vi "Write Scale.vi"(8 "error in (no error)":errorcluster, 10 "Scale":dbl, 11 "Multiplexer configuration in":refnum<class "Multiplexer configuration.lvclass">) -> (0 "error out":errorcluster, 3 "Multiplexer configuration out":refnum<class "Multiplexer configuration.lvclass">)   [LabVIEW 2021, in "Multiplexer configuration.lvclass"]
uses:
  Multiplexer configuration.lvclass
  Multiplexer configuration.lvclass/Multiplexer configuration.ctl
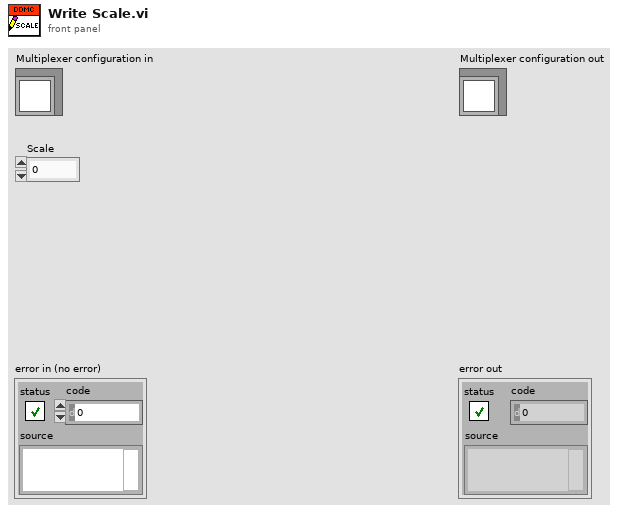
[diagram p1: front panel]
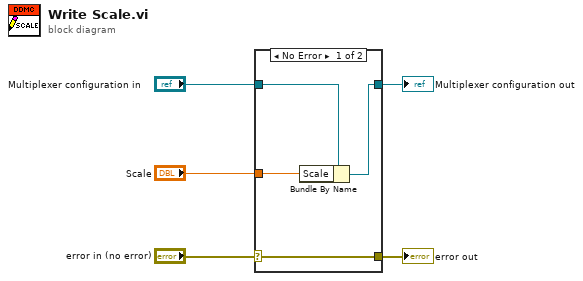
[diagram p0: block diagram]
diagram:
  n1 = case shown="No Error" "error in (no error)" {
    selector: "error in (no error)" -> [w9 w10]
    tunnel: [w9 w10] -> w4
    tunnel: [w7 w11] -> w2
    tunnel: "Multiplexer configuration in" -> [w8 w11]
    tunnel: "Scale" -> [w6 _]
    frame No Error {
      n2 = Bundle By Name(cluster=w8, "Scale"=w6) -> (w7:refnum<class "Multiplexer configuration.lvclass">)
    }
    frame Error {
    }
  }
  "error out" <- w4
  "Multiplexer configuration out" <- w2
